vi "Calc_Top.vi"(8 "Draw?":bool, 9 "Edge Points":cluster{dbl, dbl}[][](array[cluster]), 11 "picture in":picture) -> (1 "All Points":cluster{"x":dbl, "y":dbl}[][](array[cluster]), 3 "picture out":picture)   [LabVIEW 2022 SP3]
uses:
  Perspective_Globals.vi
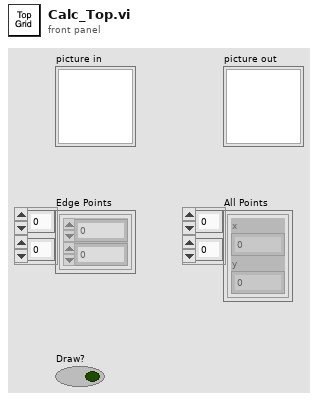
[diagram p1: front panel]
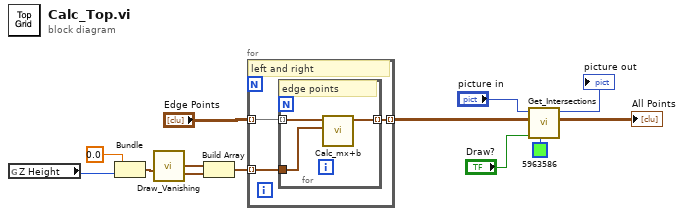
[diagram p0: block diagram]
diagram:
  n1 = global read "Perspective_Globals.vi" "Z Height"() -> (w3:i32)
  n2 = Bundle(0.0, "Z Height"=w3) -> (w1:cluster{dbl, "Z Height":i32})  [unwired: 1 in]
  n3 = call "Draw_Vanishing.vi"("point"=w1) -> ("right_line"=w5:cluster{"slope":dbl, "b":dbl, "theta":dbl}, "left_line"=w4:cluster{"slope":dbl, "b":dbl, "theta":dbl})  [unwired: 8 in, 1 out]
  n4 = Build Array(w4, w5) -> (w6:cluster{"slope":dbl, "b":dbl, "theta":dbl}[])
  n5 = for {
    tunnel: "Edge Points" -> [w16] mode=indexing
    tunnel: w6 -> [w15] mode=indexing
    tunnel: [w14] -> w8 mode=indexing
    # "left and right"
    n6 = for {
      tunnel: w16 -> [w18] mode=indexing
      tunnel: w15 -> [w19]
      tunnel: [w17] -> w14 mode=indexing
      # "edge points"
      n7 = call "Calc_mx+b.vi"("line"=w19, "point"=w18) -> ("point on line"=w17:cluster{"x":dbl, dbl})  [unwired: 9 in]
    }
  }
  n8 = call "Get_Intersections.vi"("color"=u32 5963586, "Draw?"="Draw?", "Edge Points"=w8, "picture in"="picture in") -> ("All Points"=→"All Points":cluster{"x":dbl, "y":dbl}[][], "picture out"=→"picture out":picture)  [unwired: 6 in]
